vi "Basic GUI Axis control.vi"() -> ()   [LabVIEW 2015]
panel:
  out "PosRemaining":sgl
  in  "Speed":sgl
  out "Current Position":sgl
  in  "stop":bool
  in  "Jog":bool
  in  "GoTo":bool
  in  "Setpoint":sgl
  in  "Enable Axis":bool
  in  "MintControls5560Lib.MintControllerCtrl":refnum<k7>(container)
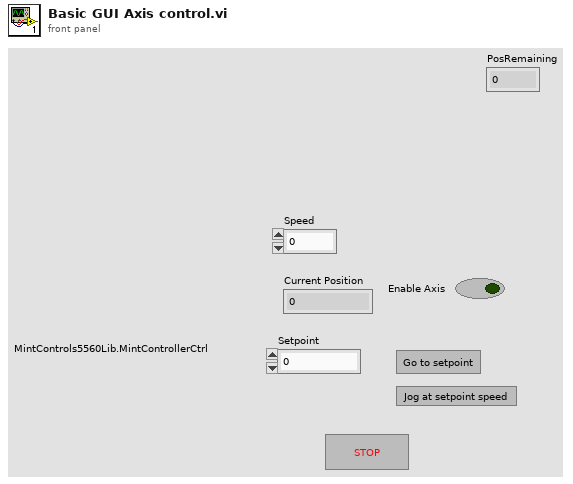
[diagram p1: front panel]
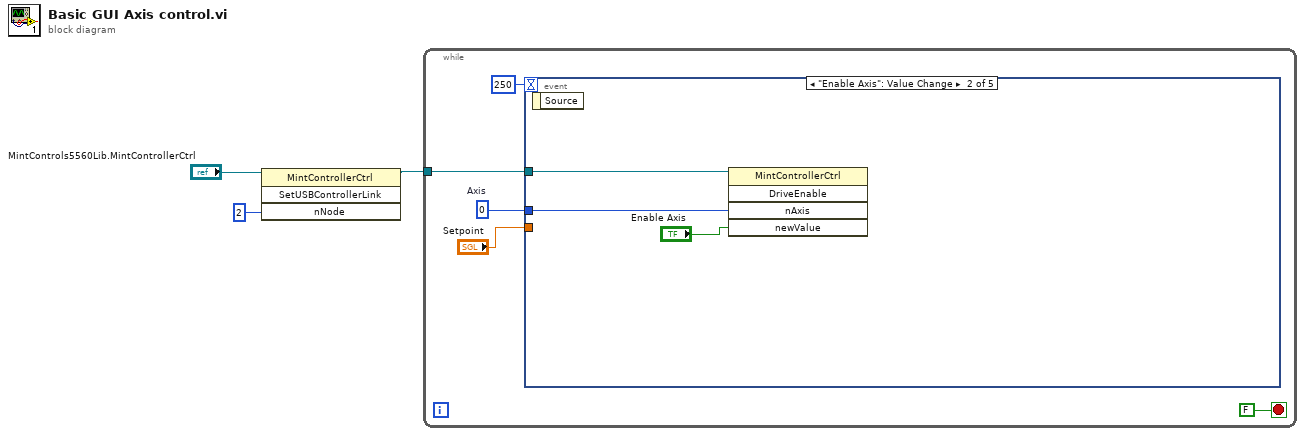
[diagram p0: block diagram]
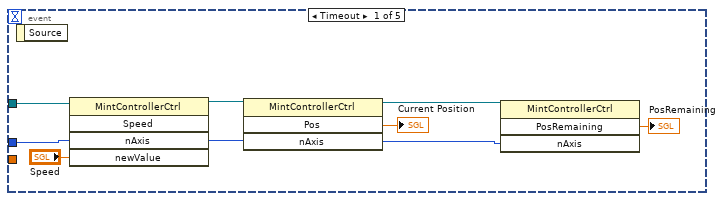
[diagram p2: hidden frame]
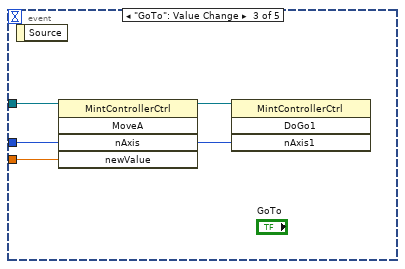
[diagram p3: hidden frame]
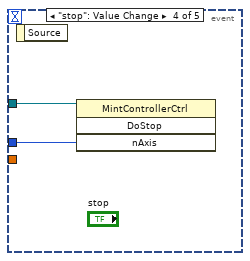
[diagram p4: hidden frame]
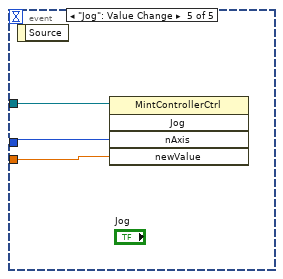
[diagram p5: hidden frame]
diagram:
  n1 = invoke class="MintControllerCtrl" method="SetUSBControllerLink"(reference="MintControls5560Lib.MintControllerCtrl", "nNode"=i16 2) -> (reference out=w1:refnum<k7>)  [unwired: 2 in, 3 out]
  n2 = while {
    tunnel: w1 -> [w8]
    stop <- FALSE stop-if-true
    w7 = i16 0  # Axis
    n3 = event shown="[1] \"Enable Axis\": Value Change" {
      selector: _ -> [_ _ _ _ _]
      dyn-events: _ -> [_ _ _ _ _]
      timeout: 250 -> [_ _ _ _ _]
      tunnel: w8 -> [w16 w20 w25 w27 w29]
      tunnel: w7 -> [w14 w18 w24 w26 w30]
      tunnel: "Setpoint" -> [_ _ w23 _ w28]
      event Timeout {
        n4 = event-data() -> ()  [unwired: 1 in, 1 out]
        n5 = invoke class="MintControllerCtrl" method="Speed"(reference=w16, "nAxis"=w14, "newValue"="Speed") -> (reference out=w15:refnum<k7>, "nAxis"=w13:i16)  [unwired: 2 in, 3 out]
        n6 = invoke class="MintControllerCtrl" method="Pos"(reference=w15, "nAxis"=w13) -> (reference out=w11:refnum<k7>, "Pos"=→"Current Position":sgl, "nAxis"=w10:i16)  [unwired: 2 in, 1 out]
        n7 = invoke class="MintControllerCtrl" method="PosRemaining"(reference=w11, "nAxis"=w10) -> ("PosRemaining"=→"PosRemaining":sgl)  [unwired: 2 in, 3 out]
      }
      event "Enable Axis": Value Change {
        n8 = event-data() -> ()  [unwired: 1 in, 1 out]
        n9 = invoke class="MintControllerCtrl" method="DriveEnable"(reference=w20, "nAxis"=w18, "newValue"="Enable Axis") -> ()  [unwired: 2 in, 5 out]
      }
      event "GoTo": Value Change {
        n10 = event-data() -> ()  [unwired: 1 in, 1 out]
        n11 = invoke class="MintControllerCtrl" method="MoveA"(reference=w25, "nAxis"=w24, "newValue"=w23) -> (reference out=w22:refnum<k7>, "nAxis"=w21:i16)  [unwired: 2 in, 3 out]
        n12 = invoke class="MintControllerCtrl" method="DoGo1"(reference=w22, "nAxis1"=w21) -> ()  [unwired: 2 in, 4 out]
      }
      event "stop": Value Change {
        n13 = event-data() -> ()  [unwired: 1 in, 1 out]
        n14 = invoke class="MintControllerCtrl" method="DoStop"(reference=w27, "nAxis"=w26) -> ()  [unwired: 2 in, 4 out]
      }
      event "Jog": Value Change {
        n15 = event-data() -> ()  [unwired: 1 in, 1 out]
        n16 = invoke class="MintControllerCtrl" method="Jog"(reference=w29, "nAxis"=w30, "newValue"=w28) -> ()  [unwired: 2 in, 5 out]
      }
    }
  }
